vi "GetObjectConfiguration.vi"(8 "ErrorIn":errorcluster, 9 "DataIn":variant, 10 "Label":string, 11 "ReferenceIn":refnum<class "AppConfigJSON.lvclass">) -> (0 "ErrorOut":errorcluster, 1 "DataOut":variant, 3 "ReferenceOut":refnum<class "AppConfigJSON.lvclass">)   [LabVIEW 2021, in "AppConfigJSON.lvclass"]
uses:
  AppConfigJSON.lvclass
  <vilib>/JDP Science/JSONtext/Config Files/Config File.lvclass/Config File.ctl
  959408aa-d2e9-4604-884c-06ccb445daab.vi
  aefc3f97-8a07-48d2-89a6-7f25208ebf9e.vi
  <vilib>/JDP Science/JSONtext/JSON text to Variant.vi
  <vilib>/JDP Science/JSONtext/Variant to JSON Text.vi
  <vilib>/JDP Science/JSONtext/Config Files/Write Config to File.vi
  <vilib>/JDP Science/JSONtext/LVClass Serializer/JSONtext LVClass Serializer.lvclass
  AppConfigJSON.lvclass/AppConfigJSON.ctl
  <vilib>/JDP Science/JSONtext/Config Files/Config File.lvclass
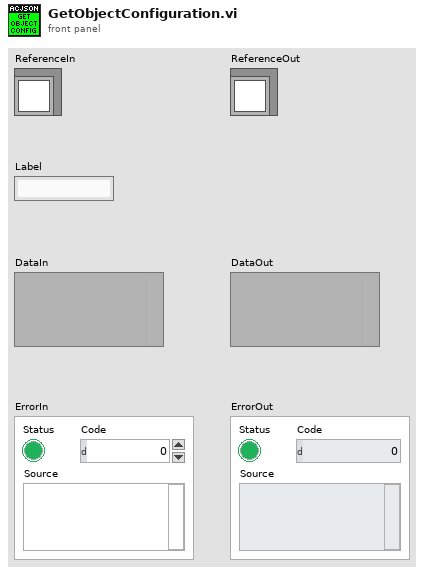
[diagram p1: front panel]
types:
  T1 = typedef "AppConfigJSON.lvclass/ObjectAttributes.ctl" = cluster{"Name":string, "ConfigFilePath":path, "Objects":T2[], "ApplicationBasePath":path, "ObjectName":string}
  T2 = typedef "IApplicationConfiguration.lvclass/ObjectDataDetails.ctl" = cluster{"ObjectName":string, "ObjectType":string, "Interfaces":T3[]}
  T3 = typedef "IApplicationConfiguration.lvclass/ObjectData.ctl" = cluster{"Label":string, "ObjectName":string, "Type":string}
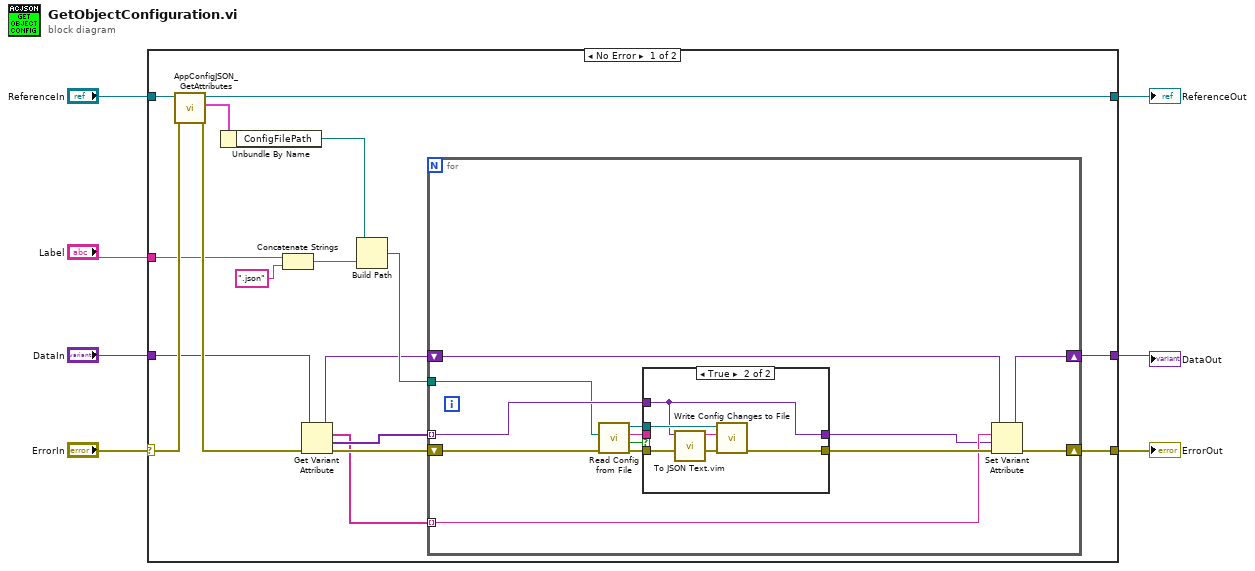
[diagram p0: block diagram]
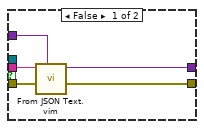
[diagram p2: hidden frame]
diagram:
  n1 = case shown="No Error" "ErrorIn" {
    selector: "ErrorIn" -> [w22 w49]
    tunnel: [w21 w49] -> w6
    tunnel: [w18 w48] -> w4
    tunnel: "ReferenceIn" -> [w19 w48]
    tunnel: "Label" -> [w8 _]
    tunnel: "DataIn" -> [w17 w47]
    tunnel: [w10 w47] -> w1
    frame No Error {
      n2 = call "AppConfigJSON_GetAttributes.vi"("ErrorIn"=w22, "ReferenceIn"=w19) -> ("ErrorOut"=w21:errorcluster, "Data"=w20:T1, "ReferenceOut"=w18:refnum<class "AppConfigJSON.lvclass">)  [unwired: 6 in, 1 out]
      n3 = Unbundle By Name(w20) -> ("ConfigFilePath"=w9:path)
      n4 = Concatenate Strings(w8, ".json" ("string")) -> (w15:string)
      n5 = Get Variant Attribute(Variant=w17, error in=w21) -> (duplicate Variant=w11:variant, names=w12:string[], values=w13:variant[])  [unwired: 2 in, 1 out]
      n6 = Build Path(base path=w9, name or relative path=w15) -> (appended path=w16:path)
      n7 = for {
        tunnel: w16 -> [w26]
        tunnel: w13 -> [w28] mode=indexing
        tunnel: w12 -> [w29] mode=indexing
        shift-right: [w35] -> _
        shift-left: w21 -> [w33]
        shift-right: [w30] -> w10
        shift-left: w11 -> [w31]
        n8 = call <vilib>:"Read Config from File.vi"("error in (no error)"=w33, "config file path"=w26) -> ("error out"=w32:errorcluster, "Template Used (file missing or corrupted)"=w24:bool, "<JSON>Config"=w25:string, "Config File"=w23:refnum<class "Config File.lvclass">)  [unwired: 6 in]
        n9 = case shown="True" w24 {
          tunnel: w28 -> [w38 w41]
          tunnel: [w37 w41] -> w27
          tunnel: [w40 w44] -> w34
          tunnel: w25 -> [w36 _]
          tunnel: w32 -> [w39 w46]
          tunnel: w23 -> [_ w42]
          frame False {
            n10 = call "From JSON Text.vim"("Data Type and Default Value"=w38, "error in (no error)"=w39, "JSON"=w36) -> ("error out"=w40:errorcluster, "Data out"=w37:variant)  [unwired: 7 in]
          }
          frame True {
            n11 = call "To JSON Text.vim"("error in (no error)"=w46, "Anything"=w41) -> ("error out"=w45:errorcluster, "<JSON>"=w43:string)  [unwired: 8 in]
            n12 = call <vilib>:"Write Config Changes to File.vi"("error in (no error)"=w45, "New Config"=w43, "Config File in"=w42) -> ("error out"=w44:errorcluster)  [unwired: 5 in, 3 out]
          }
        }
        n13 = Set Variant Attribute(Variant=w31, name=w29, value=w27, error in=w34) -> (Variant out=w30:variant, error out=w35:errorcluster)  [unwired: 1 out]
      }
    }
    frame Error {
    }
  }
  "ErrorOut" <- w6
  "ReferenceOut" <- w4
  "DataOut" <- w1
